vi "Global - RT Channels.vi"() -> ()   [LabVIEW 2018]
panel:
  in  "Pump 5 Running":refnum<k21>="ni.var.io://192.168.1.2/EtherCAT/HPU/04DI/02AtSpeedMtr5"
  in  "Pump 4 Running":refnum<k21>="ni.var.io://192.168.1.2/EtherCAT/HPU/04DI/08AtSpeedMtr4"
  in  "Pump 3 Running":refnum<k21>="ni.var.io://192.168.91.21/01DI/16 FB AV1O"
  in  "Pump 2 Running":refnum<k21>="ni.var.io://192.168.91.21/01DI/16 FB AV1O"
  in  "Pump 1 Running":refnum<k21>="ni.var.io://192.168.91.21/01DI/16 FB AV1O"
  in  "Stop Cool Fan":refnum<k21>="ni.var.io://192.168.1.2/EtherCAT/HPU/05DO/06StopCoolFan"
  in  "Run Cool Fan":refnum<k21>="ni.var.io://192.168.1.2/EtherCAT/HPU/05DO/05RunCoolFan"
  in  "Run Pump 5":refnum<k21>="ni.var.io://192.168.1.2/EtherCAT/HPU/05DO/04RunMotor5"
  in  "Run Pump 4":refnum<k21>="ni.var.io://192.168.1.2/EtherCAT/HPU/05DO/03RunMotor4"
  in  "Run Pump 3":refnum<k21>="ni.var.io://192.168.1.2/EtherCAT/HPU/05DO/02RunMotor3"
  in  "Run Pump 2":refnum<k21>="ni.var.io://192.168.1.2/EtherCAT/HPU/05DO/01RunMotor2"
  in  "Run Pump 1":refnum<k21>="ni.var.io://192.168.1.2/EtherCAT/HPU/05DO/00RunMotor1"
  # "Extension HPU"
  # "DO"
  # "DI"
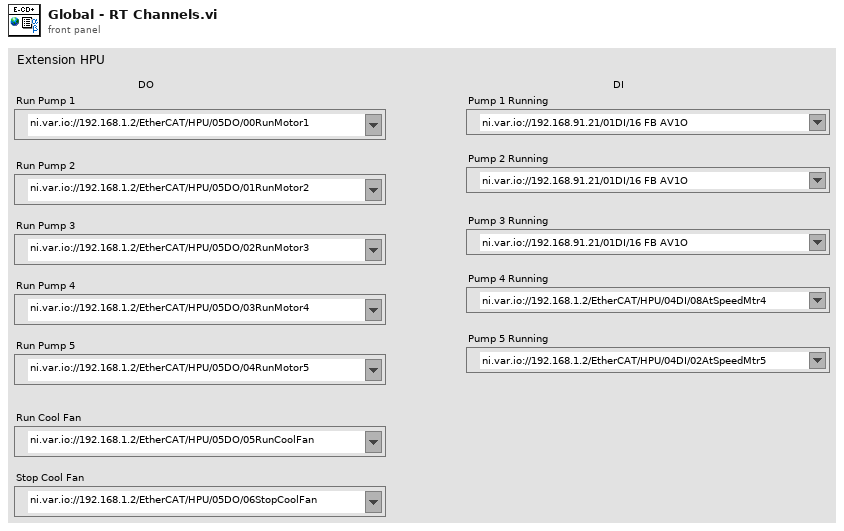
[diagram p1: front panel]
diagram:
